vi "Get_run_info.vi"(1 "Run Info Cluster In":T1={"Set Point (*C)"=0, "Field (uT)"=0.0, "Soak Time (min)"=30, "Atmosphere"="1", "User"="", "Note"="", "email address"="", "Email"=FALSE, "Field on (*C)"=0.0, "Field off (*C)"=0.0, "Enable field"=FALSE, "log fO2 rel. IW/IM"=0.0}) -> (0 "Run Info Cluster Out":T1={"Set Point (*C)"=0, "Field (uT)"=0.0, "Soak Time (min)"=30, "Atmosphere"="1", "User"="", "Note"="", "email address"="", "Email"=FALSE, "Field on (*C)"=0.0, "Field off (*C)"=0.0, "Enable field"=FALSE, "log fO2 rel. IW/IM"=0.0})   [LabVIEW 2009]
doc: "Displays window to gather information about user and run conditions.\nOutput is bundled cluster with:\n1) Use DB boolean\n2) DB User ID\n3) non-DB User Name\n4) Field on/off boolean\n5) Field magnitude\n6) Set point\n7) Soak time\n8) Atmosphere flag\n9) Note"
panel:
  in  "Abort":bool
  in  "Continue":bool
  # "Run Information"
  # "User Information"
  # "User Information"
  # "Run Information"
  # "Field (uT)"
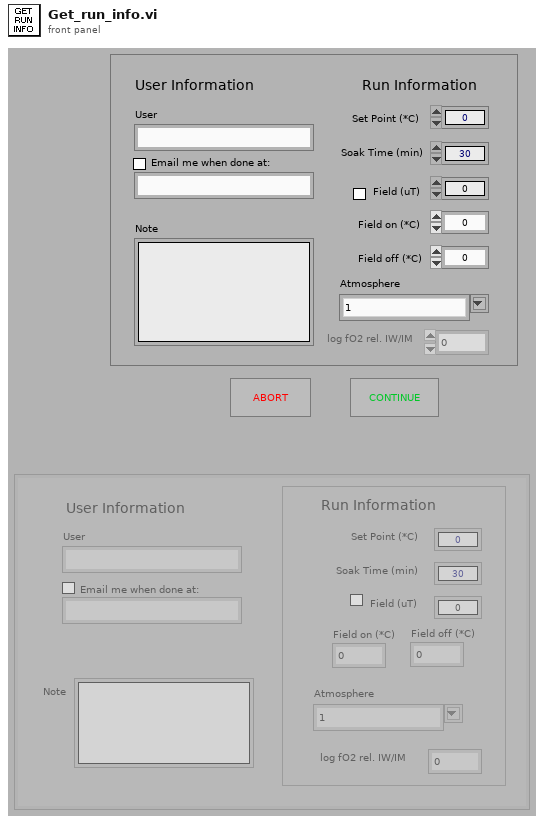
[diagram p1: front panel]
types:
  T1 = cluster{"Set Point (*C)":u32, "Field (uT)":dbl, "Soak Time (min)":u32, "Atmosphere":string, "User":string, "Note":string, "email address":string, "Email":bool, "Field on (*C)":dbl, "Field off (*C)":dbl, "Enable field":bool, "log fO2 rel. IW/IM":dbl}
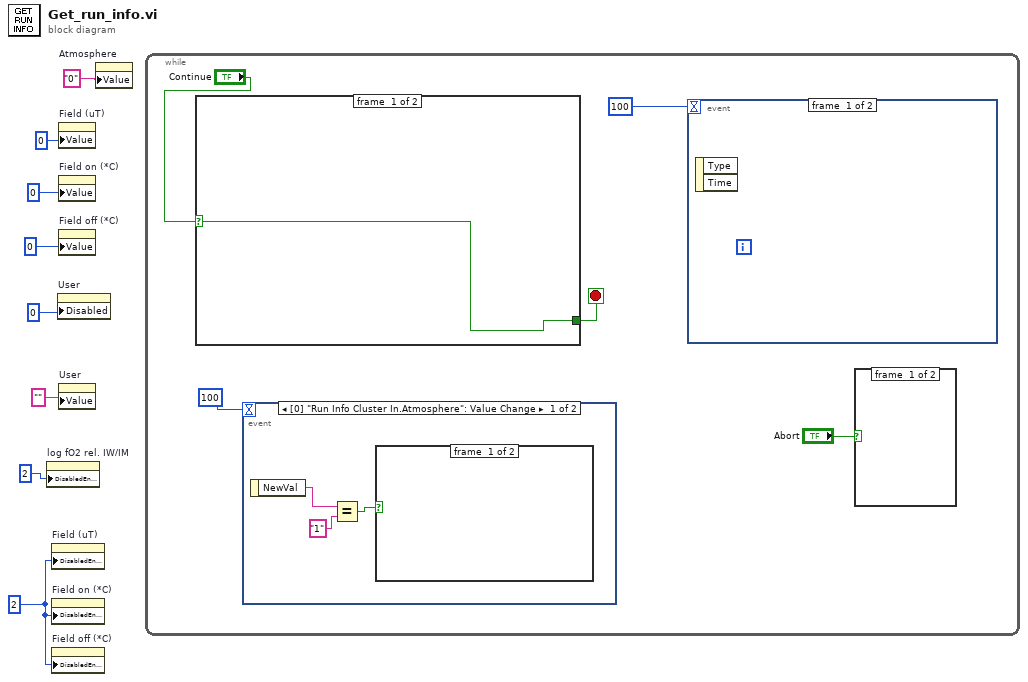
[diagram p0: block diagram]
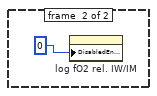
[diagram p2: hidden frame]
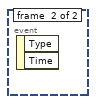
[diagram p3: hidden frame]
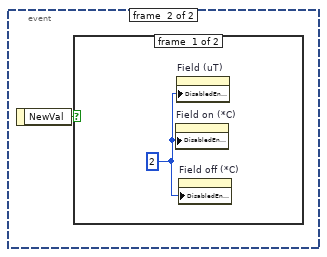
[diagram p4: hidden frame]
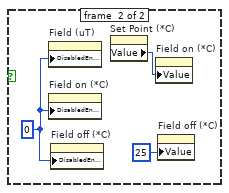
[diagram p5: hidden frame]
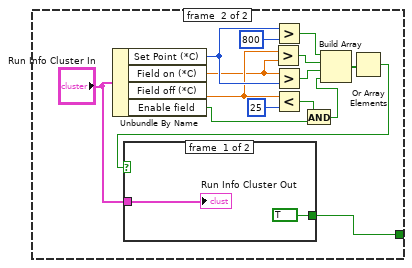
[diagram p6: hidden frame]
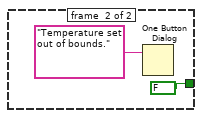
[diagram p7: hidden frame]
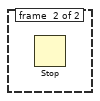
[diagram p8: hidden frame]
diagram:
  w1 = 2
  n1 = property on="log fO2 rel. IW/IM" class="DigNum (strict)"("DisabledEnum"=2) -> ()  [unwired: 2 in, 2 out]
  n2 = property on="Field (uT)" class="DigNum (strict)"("DisabledEnum"=w1) -> ()  [unwired: 2 in, 2 out]
  n3 = property on="Field on (*C)" class="DigNum (strict)"("DisabledEnum"=w1) -> ()  [unwired: 2 in, 2 out]
  n4 = property on="Field off (*C)" class="DigNum (strict)"("DisabledEnum"=w1) -> ()  [unwired: 2 in, 2 out]
  n5 = property on="User" class="Str"("Disabled"=u8 0) -> ()  [unwired: 2 in, 2 out]
  n6 = property on="Field (uT)" class="DigNum (strict)"("Value"=0) -> ()  [unwired: 2 in, 2 out]
  n7 = property on="Field on (*C)" class="DigNum (strict)"("Value"=0) -> ()  [unwired: 2 in, 2 out]
  n8 = property on="Field off (*C)" class="DigNum (strict)"("Value"=0) -> ()  [unwired: 2 in, 2 out]
  n9 = property on="User" class="Str"("Value"="") -> ()  [unwired: 2 in, 2 out]
  n10 = property on="Atmosphere" class="CmbBox"("Value"="0") -> ()  [unwired: 2 in, 2 out]
  n11 = while {
    stop <- w11 stop-if-true
    n12 = case shown="True" "Continue" {
      selector: "Continue" -> [w23 _]
      tunnel: [w23 w37] -> w11
      frame #0 {
      }
      frame #1 {
        n13 = Unbundle By Name("Run Info Cluster In") -> ("Set Point (*C)"=w34:u32, "Field on (*C)"=w27:dbl, "Field off (*C)"=w28:dbl, "Enable field"=w25:bool)
        n14 = Greater?(x=w28, y=w27) -> (0:w29:bool)
        n15 = Greater?(x=w34, y=u32 800) -> (0:w33:bool)
        n16 = Greater?(x=w27, y=w34) -> (0:w32:bool)
        n17 = Less?(x=w28, y=25) -> (x < y?=w26:bool)
        n18 = And(x=w26, y=w25) -> (x .and. y?=w24:bool)
        n19 = Build Array(w33, w29, w32, w24) -> (w31:bool[])
        n20 = Or Array Elements(Boolean array=w31) -> (logical OR=w30:bool)
        n21 = case shown="False" w30 {
          tunnel: [TRUE FALSE] -> w37
          tunnel: "Run Info Cluster In" -> [w39 _]
          frame #0 {
            "Run Info Cluster Out" <- w39
          }
          frame #1 {
            n22 = One Button Dialog(message="Temperature set out of bounds.") -> ()  [unwired: 2 out]
          }
        }
      }
    }
    n23 = event shown="[0] \"Run Info Cluster In.Atmosphere\": Value Change" {
      selector: _ -> [_ _]
      dyn-events: _ -> [_ _]
      timeout: 100 -> [_ _]
      event #0 {
        n24 = event-data() -> ("NewVal"=w16:string)  [unwired: 1 in]
        n25 = Equal?(x=w16, y="1") -> (x = y?=w14:bool)
        n26 = case shown="True" w14 {
          frame #0 {
          }
          frame #1 {
            n27 = property on="log fO2 rel. IW/IM" class="DigNum (strict)"("DisabledEnum"=0) -> ()  [unwired: 2 in, 2 out]
          }
        }
      }
      event #1 {
        n28 = event-data() -> ()  [unwired: 1 in, 2 out]
      }
    }
    n29 = event shown="[1] \"Run Info Cluster In.Enable field\": Value Change" {
      selector: _ -> [_ _]
      dyn-events: _ -> [_ _]
      timeout: 100 -> [_ _]
      event #0 {
        n30 = event-data() -> ()  [unwired: 1 in, 2 out]
      }
      event #1 {
        n31 = event-data() -> ("NewVal"=w18:bool)  [unwired: 1 in]
        n32 = case shown="True" w18 {
          frame #0 {
            w19 = 2
            n33 = property on="Field on (*C)" class="DigNum (strict)"("DisabledEnum"=w19) -> ()  [unwired: 2 in, 2 out]
            n34 = property on="Field (uT)" class="DigNum (strict)"("DisabledEnum"=w19) -> ()  [unwired: 2 in, 2 out]
            n35 = property on="Field off (*C)" class="DigNum (strict)"("DisabledEnum"=w19) -> ()  [unwired: 2 in, 2 out]
          }
          frame #1 {
            w22 = 0
            n36 = property on="Field (uT)" class="DigNum (strict)"("DisabledEnum"=w22) -> ()  [unwired: 2 in, 2 out]
            n37 = property on="Field on (*C)" class="DigNum (strict)"("DisabledEnum"=w22) -> ()  [unwired: 2 in, 2 out]
            n38 = property on="Field off (*C)" class="DigNum (strict)"("DisabledEnum"=w22) -> ()  [unwired: 2 in, 2 out]
            n39 = property on="Set Point (*C)" class="DigNum (strict)"() -> ("Value"=w21:u32)  [unwired: 2 in, 2 out]
            n40 = property on="Field on (*C)" class="DigNum (strict)"("Value"=w21) -> ()  [unwired: 2 in, 2 out]
            n41 = property on="Field off (*C)" class="DigNum (strict)"("Value"=25) -> ()  [unwired: 2 in, 2 out]
          }
        }
      }
    }
    n42 = case shown="True" "Abort" {
      frame #0 {
      }
      frame #1 {
        n43 = Stop() -> ()  [unwired: 1 out]
      }
    }
  }
